vi "Script Version VI.vi"(8 "error in (no error)":errorcluster, 9 "Commit Reference":string, 10 "Version String":string, 11 "Library Refnum":refnum<vi>) -> (0 "error out":errorcluster, 1 "Library Description":string, 2 "Added Version VI":bool, 3 "Library Refnum out":refnum<vi>)   [LabVIEW 2019]
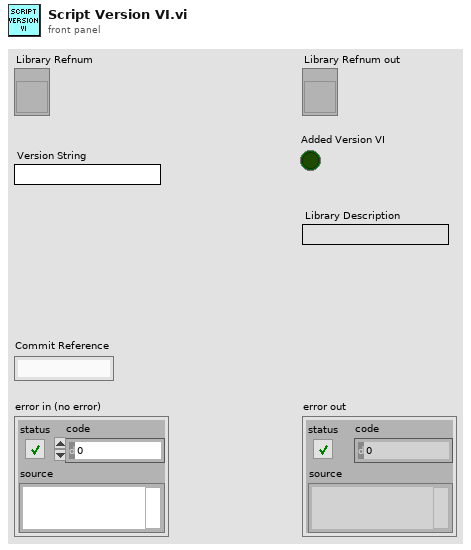
[diagram p1: front panel]
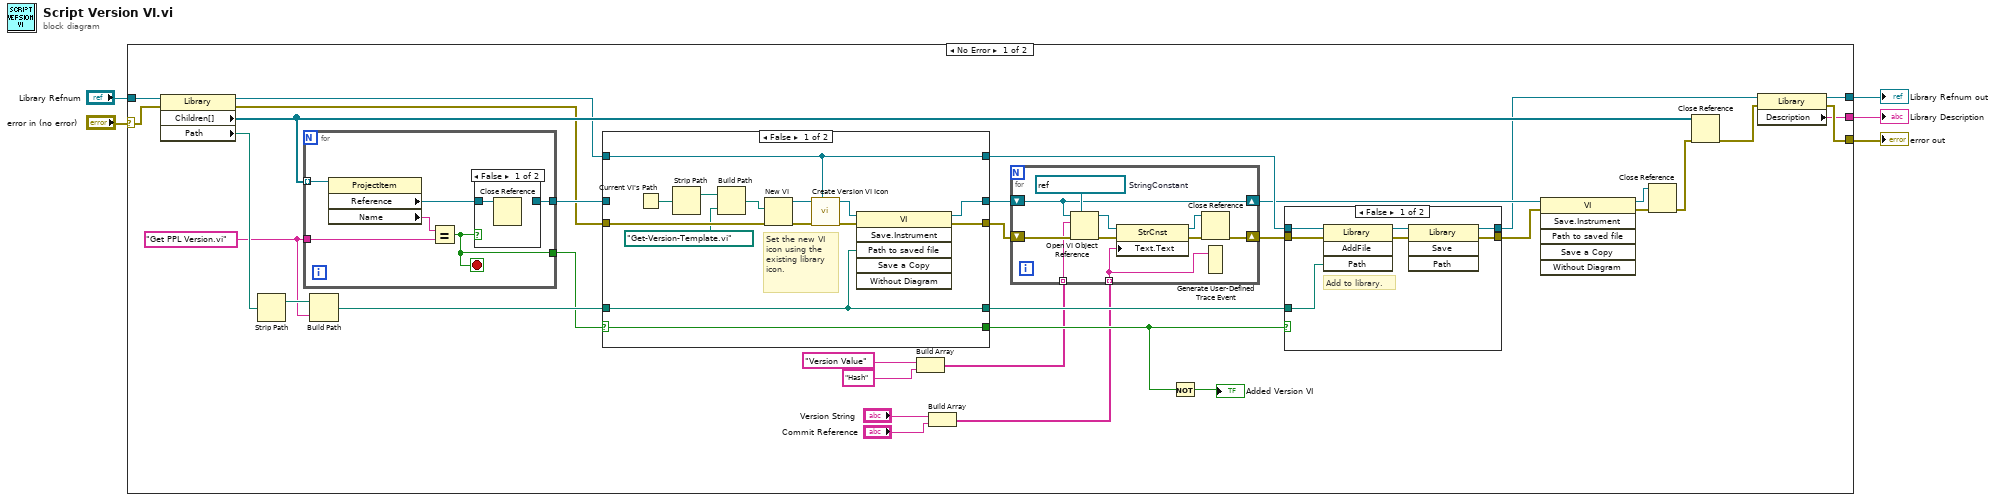
[diagram p0: block diagram]
diagram:
  n1 = case shown="No Error" "error in (no error)" {
    selector: "error in (no error)" -> [w13 w87]
    tunnel: "Library Refnum" -> [w34 w86]
    tunnel: [w8 w87] -> w4
    tunnel: [w10 w86] -> w3
    tunnel: [w7 _] -> w1
    frame No Error {
      w36 = "Get PPL Version.vi" ("name or relative path")
      n2 = property class="Library"(reference=w34, error in=w13) -> (reference out=w29:refnum<vi>, error out=w31:errorcluster, "Children[]"=w32:refnum<vi>[], "Path"=w38:path)
      n3 = Strip Path(path=w38) -> (stripped path=w37:path)  [unwired: 1 out]
      n4 = for {
        tunnel: w32 -> [w45] mode=indexing
        tunnel: w36 -> [w44]
        tunnel: [w42] -> w12
        tunnel: [w41] -> w33
        stop <- w42 stop-if-true
        n5 = property class="ProjectItem"(reference=w45) -> ("Reference"=w43:refnum<vi>, "Name"=w40:string)  [unwired: 1 in, 2 out]
        n6 = Equal?(x=w40, y=w44) -> (x = y?=w42:bool)
        n7 = case shown="False" w42 {
          tunnel: w43 -> [w46 w47]
          tunnel: [_ w47] -> w41
          frame False {
            n8 = Close Reference(reference=w46) -> ()  [unwired: 1 in, 1 out]
          }
          frame True {
          }
        }
      }
      n9 = Build Path(base path=w37, name or relative path=w36) -> (appended path=w28:path)
      n10 = case shown="False" w12 {
        selector: w12 -> [w74 w81]
        tunnel: w33 -> [_ w85]
        tunnel: w31 -> [w80 w84]
        tunnel: [w78 w85] -> w24
        tunnel: [w76 w84] -> w30
        tunnel: w29 -> [w67 w83]
        tunnel: [w67 w83] -> w26
        tunnel: w28 -> [w75 w82]
        tunnel: [w75 w82] -> w25
        tunnel: [w74 w81] -> w20
        frame False {
          # "Set the new VI icon using the existing library icon."
          n11 = Current VI's Path() -> (path=w72:path)
          n12 = Strip Path(path=w72) -> (stripped path=w71:path)  [unwired: 1 out]
          n13 = Build Path(base path=w71, name or relative path=path "Get-Version-Template.vi" ("template")) -> (appended path=w70:path)
          n14 = New VI(8:w80, 10:w70) -> (0:w68:errorcluster, 3:w69:refnum<vi>)  [unwired: 5 in]
          n15 = call "Create Version VI Icon.vi"("Library Ref"=w67, "error in (no error)"=w68, "VI Ref"=w69) -> ("error out"=w77:errorcluster, "VI out"=w79:refnum<vi>)  [unwired: 7 in]
          n16 = invoke class="VI" method="Save.Instrument"(reference=w79, error in=w77, "Path to saved file"=w75) -> (reference out=w78:refnum<vi>, error out=w76:errorcluster)  [unwired: 3 in, 4 out]
        }
        frame True {
        }
      }
      n17 = Build Array("Version Value" ("name/order"), "Hash" ("name/order")) -> (w14:string[])
      n18 = Build Array("Version String", "Commit Reference") -> (w19:string[])
      n19 = for {
        tunnel: w19 -> [w48] mode=indexing
        shift-right: [w51] -> w23
        shift-left: w30 -> [w52]
        shift-right: [w50] -> w15
        shift-left: w24 -> [w50]
        tunnel: w14 -> [w49] mode=indexing
        w57 = refnum<vi> refnum  # StringConstant
        n20 = Open VI Object Reference(7:w57, 8:w52, 10:w49, 11:w50) -> (0:w56:errorcluster, 3:w53:refnum<vi>)
        n21 = property class="StrCnst"(reference=w53, error in=w56, "Text.Text"=w48) -> (reference out=w55:refnum<vi>, error out=w54:errorcluster)
        n22 = Close Reference(reference=w55, error in (no error)=w54) -> (error out=w51:errorcluster)
        n23 = Generate User-Defined Trace Event(2:w48) -> ()  [unwired: 1 in]
      }
      n24 = Not(x=w20) -> (.not. x?=→"Added Version VI":bool)
      n25 = case shown="False" w20 {
        tunnel: w23 -> [w64 w65]
        tunnel: w26 -> [w62 w66]
        tunnel: w25 -> [w61 _]
        tunnel: [w60 w65] -> w22
        tunnel: [w58 w66] -> w11
        frame False {
          # "Add to library."
          n26 = invoke class="Library" method="AddFile"(reference=w62, error in=w64, "Path"=w61) -> (reference out=w59:refnum<vi>, error out=w63:errorcluster)  [unwired: 1 in, 2 out]
          n27 = invoke class="Library" method="Save"(reference=w59, error in=w63) -> (reference out=w58:refnum<vi>, error out=w60:errorcluster)  [unwired: 2 in, 2 out]
        }
        frame True {
        }
      }
      n28 = invoke class="VI" method="Save.Instrument"(reference=w15, error in=w22) -> (reference out=w35:refnum<vi>, error out=w39:errorcluster)  [unwired: 4 in, 4 out]
      n29 = Close Reference(reference=w35, error in (no error)=w39) -> (error out=w21:errorcluster)
      n30 = Close Reference(reference=w32, error in (no error)=w21) -> (error out=w9:errorcluster)
      n31 = property class="Library"(reference=w11, error in=w9) -> (reference out=w10:refnum<vi>, error out=w8:errorcluster, "Description"=w7:string)
    }
    frame Error {
    }
  }
  "Library Refnum out" <- w3
  "error out" <- w4
  "Library Description" <- w1
